vi "create_image_message.vi"(8 "error in (no error)":errorcluster, 9 "images":path[](array[path]), 10 "text":string[](array[string]), 11 "role":string="user") -> (0 "error out":errorcluster, 3 "message_text out":refnum<class "message_image.lvclass">)   [LabVIEW 2020, in "message_image.lvclass"]
uses:
  message_image.lvclass
  message.ctl
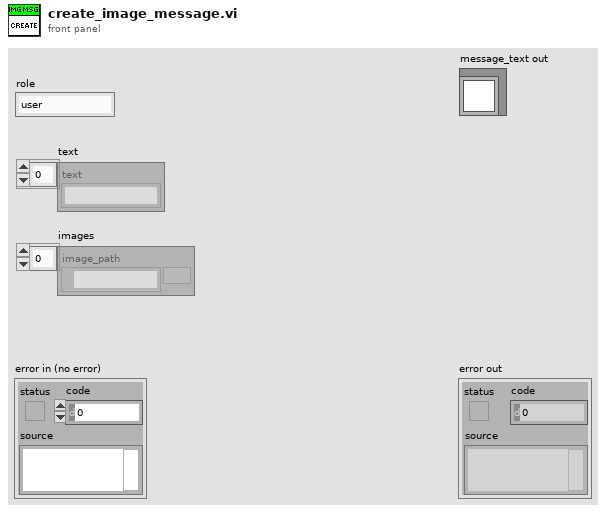
[diagram p1: front panel]
types:
  T1 = typedef "message_image.lvclass/message.ctl" = cluster{"role":string, "content_text":string[], "content_images":path[]}
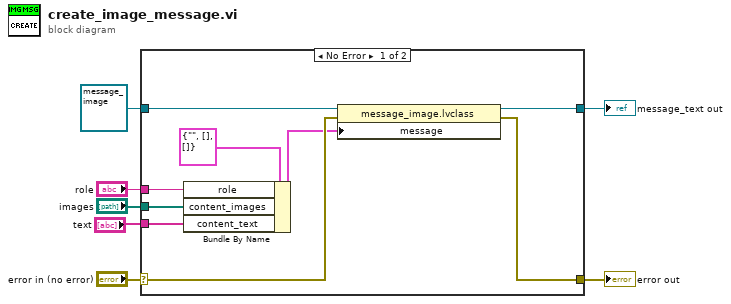
[diagram p0: block diagram]
diagram:
  n1 = case shown="No Error" "error in (no error)" {
    selector: "error in (no error)" -> [w14 w18]
    tunnel: [w13 w18] -> w6
    tunnel: [w15 w17] -> w4
    tunnel: refnum<class "message_image.lvclass"> refnum ("message_text in") -> [w16 w17]
    tunnel: "images" -> [w9 _]
    tunnel: "role" -> [w10 _]
    tunnel: "text" -> [w8 _]
    frame No Error {
      n2 = Bundle By Name(cluster=T1 {"role"="", "content_text"=[], "content_images"=[]} ("message"), "role"=w10, "content_images"=w9, "content_text"=w8) -> (w11:T1)
      n3 = property class="message_image.lvclass"(reference=w16, error in=w14, "message"=w11) -> (reference out=w15:refnum<class "message_image.lvclass">, error out=w13:errorcluster)
    }
    frame Error {
    }
  }
  "error out" <- w6
  "message_text out" <- w4
